vi "Reg2.vi"() -> ()   [LabVIEW 2010]
uses:
  <instrlib>/niScope/Controls/niScope vertical coupling.ctl
  <instrlib>/niScope/Controls/niScope trigger coupling.ctl
  <instrlib>/niScope/Controls/niScope trigger slope.ctl
  <instrlib>/niScope/Controls/niScope trigger source.ctl
  <instrlib>/niScope/Configure/Trigger/niScope Configure Trigger Immediate.vi
  <instrlib>/niScope/Acquire/niScope Multi Read WDT.vi
panel:
  out "Table":string[][](table)
  out "wfm info":T1(array[cluster]) {"reserved2" format="%.2f"; "reserved1" format="%.2f"; "offset" format="%^.3e"; "gain" format="%^.3e"; "xIncrement" format="%^.3e"; "relativeInitialX" format="%^.3e"; "absoluteInitialX" format="%^.3e"}
  out "error out":errorcluster
  out "time":timestamp
  out "Waveform Graph":waveform(i16)[](graph)
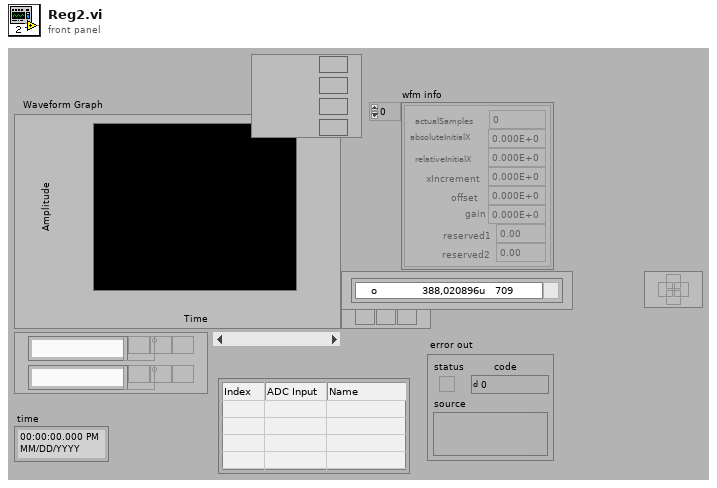
[diagram p1: front panel]
types:
  T1 = cluster{"actualSamples":i32, "absoluteInitialX":dbl, "relativeInitialX":dbl, "xIncrement":dbl, "offset":dbl, "gain":dbl, "reserved1":dbl, "reserved2":dbl}[]
  T2 = cluster{"name":enum16{"sync", "phase_a", "phase_b", "phase_c", "ground"}, "num":i32}[]
  T3 = typedef "niScope trigger source.ctl" = string
  T4 = typedef "niScope trigger slope.ctl" = i32
  T5 = typedef "niScope trigger coupling.ctl" = u16
  T6 = typedef "niScope vertical coupling.ctl" = i32
  T7 = enum16{"sync", "phase_a", "phase_b", "phase_c", "ground"}
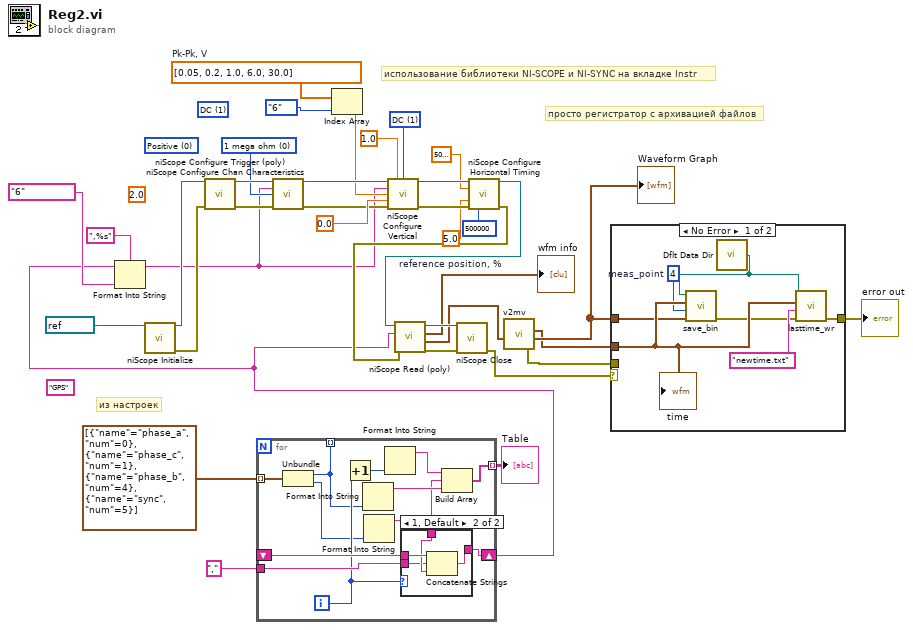
[diagram p0: block diagram]
diagram:
  w17 = dbl[] [0.05, 0.2, 1.0, 6.0, 30.0]  # Pk-Pk, V
  (unwired) 2.0 ("trigger level")
  (unwired) T4 0 items=["Positive", "Negative"] ("trigger slope")
  (unwired) T5 1 items=["AC"=0, "DC"=1, "HF Reject"=3, "LF Reject"=4, "AC Plus HF Reject"=1001] ("trigger coupling")
  w20 = u32 0 items=["1 mega ohm"=0, "50 ohms"=2] ("input impedance")
  w27 = 5.0  # reference position, %
  w32 = T6 1 items=["AC", "DC", "Ground"] ("vertical coupling")
  (unwired) "GPS"
  # "просто регистратор с архивацией файлов"
  # "из настроек"
  # "использование библиотеки NI-SCOPE и NI-SYNC на вкладке Instr"
  n1 = call <instrlib>:"niScope Initialize.vi"("resource name"=refnum<k15> "ADC") -> ("instrument handle"=w33:refnum<k15>, "error out"=w25:errorcluster)  [unwired: 13 in]
  n2 = call-poly <instrlib>:"niScope Configure Trigger (poly).vi"("instrument handle"=w33, "error in"=w25) -> ("instrument handle out"=w24:refnum<k15>, "error out"=w23:errorcluster)  [unwired: 12 in]
  n3 = for {
    tunnel: [w39] -> _ mode=indexing
    tunnel: [w47] -> w12 mode=indexing
    shift-right: [w45] -> w9
    shift-left: _ -> [w46]
    tunnel: "," -> [w43]
    tunnel: T2 [{"name"=enum."phase_a", "num"=0}, {"name"=enum."phase_c", "num"=1}, {"name"=enum."phase_b", "num"=4}, {"name"=enum."sync", "num"=5}] -> [w41] mode=indexing
    i -> [w42]
    n4 = Unbundle(w41) -> ("name"=w39:T7, "num"=w40:i32)
    n5 = Increment(x=w42) -> (x+1=w38:i32)
    n6 = Format Into String(w39) -> (resulting string=w48:string)  [unwired: 3 in, 1 out]
    n7 = Format Into String(w40) -> (resulting string=w44:string)  [unwired: 3 in, 1 out]
    n8 = Format Into String(w38) -> (resulting string=w49:string)  [unwired: 3 in, 1 out]
    n9 = case shown="1, Default" w42 {
      tunnel: w46 -> [_ w54]
      tunnel: [w50 w53] -> w45
      tunnel: w44 -> [w50 w52]
      tunnel: w43 -> [_ w51]
      frame 0 {
      }
      frame 1, Default {
        n10 = Concatenate Strings(w54, w51, w52) -> (w53:string)
      }
    }
    n11 = Build Array(w49, w44, w48) -> (w47:string[])
  }
  "Table" <- w12
  n12 = Format Into String(format string=",%s", initial string=w9, T3 "6" ("trigger source")) -> (resulting string=w8:string)  [unwired: 1 in, 1 out]
  n13 = call <instrlib>:"niScope Configure Chan Characteristics.vi"("instrument handle"=w24, "channels"=w8, "input impedance"=w20, "error in"=w23) -> ("instrument handle out"=w21:refnum<k15>, "error out"=w22:errorcluster)  [unwired: 10 in]
  n14 = Index Array(array=w17, index=enum16{"1/20", "1/5", "1", "6", "30"}."6") -> (element=w15:dbl)
  n15 = call <instrlib>:"niScope Configure Vertical.vi"("instrument handle"=w21, "probe attenuation"=1.0, "vertical coupling"=w32, "channels"=w8, "vertical range"=w15, "vertical offset"=0.0, "error in"=w22) -> ("instrument handle out"=w34:refnum<k15>, "error out"=w35:errorcluster)  [unwired: 7 in]
  n16 = call <instrlib>:"niScope Configure Horizontal Timing.vi"("instrument handle"=w34, "min sample rate"=5000000.0, "reference position"=w27, "error in"=w35, "min record length"=500000) -> ("instrument handle out"=w28:refnum<k15>, "error out"=w29:errorcluster)  [unwired: 9 in]
  n17 = call-poly <instrlib>:"niScope Read (poly).vi"("error in"=w29, "channels"=w9, "instrument handle"=w28) -> ("error out"=w36:errorcluster, "wfm"=w13:waveform(dbl)[], "wfm info"=→"wfm info":T1, "instrument handle out"=w37:refnum<k15>)  [unwired: 5 in]
  n18 = call <instrlib>:"niScope Close.vi"("instrument handle"=w37, "error in"=w36) -> ("error out"=w4:errorcluster)  [unwired: 13 in]
  n19 = call "v2mv.vi"("ArrayIn"=w13) -> ("error out"=w1:errorcluster, "ArrayOut"=w5:waveform(i16)[], "t0"=w2:timestamp)  [unwired: 4 in]
  "Waveform Graph" <- w5
  n20 = case shown="No Error" w4 {
    selector: w4 -> [_ w62]
    tunnel: [w61 w62] -> w3
    tunnel: w2 -> [w59 _]
    tunnel: w5 -> [w58 _]
    tunnel: w1 -> [_ _]
    frame No Error {
      w56 = 4  # meas_point
      n21 = call <vilib>:"Dflt Data Dir.vi"() -> ("App:Default Data Directory"=w55:path)
      n22 = call "save_bin.vi"("SigArray"=w58, "DevNo"=w56, "timestamp"=w59, "start path"=w55) -> ("error out"=w57:errorcluster)  [unwired: 3 in, 1 out]
      n23 = call "lasttime_wr.vi"("error in"=w57, "name"="newtime.txt" ("name or relative path"), "time stamp"=w59, "start Path"=w55) -> ("error out"=w61:errorcluster)  [unwired: 2 in, 1 out]
      "time" <- w59
    }
    frame Error {
    }
  }
  "error out" <- w3
